vi "SMC Control Message.vi"   [LabVIEW 2010]
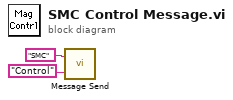
[diagram p0: block diagram]
diagram:
  n1 = call "Message Send.vi"("Message"="Control", "Destination"="SMC") -> ()
